vi "Weighted Average.vi"(1 "WeightB":dbl, 2 "WeightA":dbl, 3 "NumberB":dbl[](array[numeric]), 4 "NumberA":dbl[](array[numeric])) -> (0 "Avg":dbl[](array[numeric]))   [LabVIEW 2009]
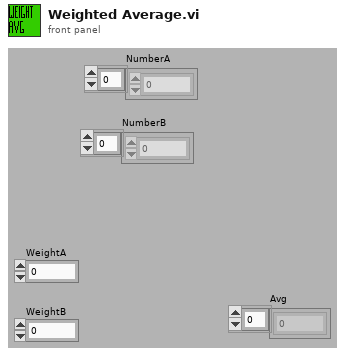
[diagram p1: front panel]
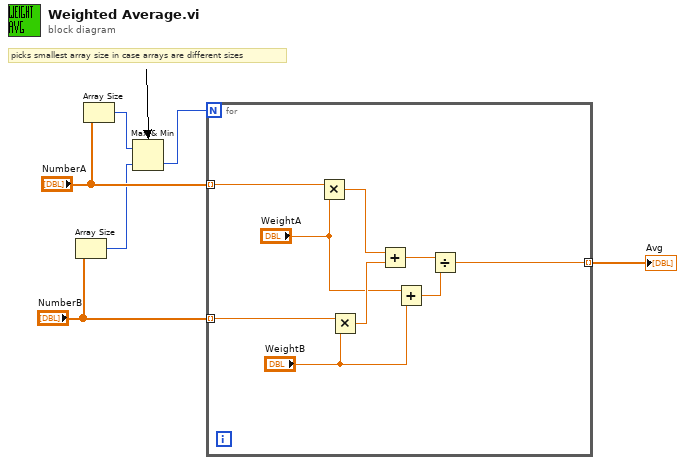
[diagram p0: block diagram]
diagram:
  # "picks smallest array size in case arrays are different sizes"
  n1 = Array Size(array="NumberB") -> (size(s)=w2:i32)
  n2 = Array Size(array="NumberA") -> (size(s)=w3:i32)
  n3 = Max & Min(x=w3, y=w2) -> (min(x,y)=w1:i32)  [unwired: 1 out]
  n4 = for {
    N: w1 -> [_]
    tunnel: [w9] -> w6 mode=indexing
    tunnel: "NumberA" -> [w8] mode=indexing
    tunnel: "NumberB" -> [w7] mode=indexing
    n5 = Multiply(x=w8, y="WeightA") -> (x*y=w15:dbl)
    n6 = Multiply(x=w7, y="WeightB") -> (x*y=w14:dbl)
    n7 = Add(x=w15, y=w14) -> (x+y=w13:dbl)
    n8 = Add(x="WeightA", y="WeightB") -> (x+y=w10:dbl)
    n9 = Divide(x=w13, y=w10) -> (x/y=w9:dbl)
  }
  "Avg" <- w6
